vi "Dequeue.vi"(8 "error in (no error)":errorcluster, 11 "Queue In":T1) -> (0 "error out":errorcluster, 1 "Variant":variant, 2 "String":string, 3 "Queue Out":T1)   [LabVIEW 2023, in "Internal Communication.lvlib"]
uses:
  Internal Communication.lvlib
  Controls/Queue.ctl
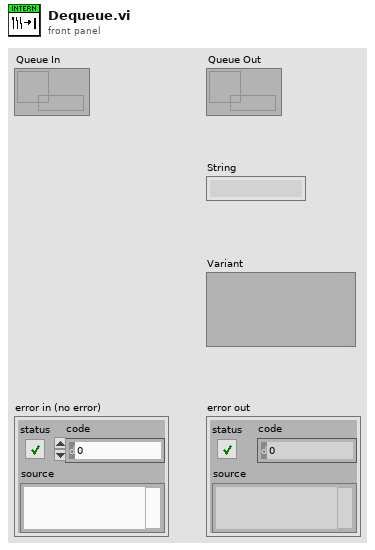
[diagram p1: front panel]
types:
  T1 = typedef "Queue.ctl" = refnum<queue>
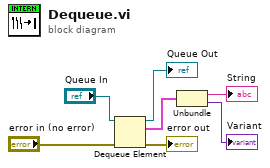
[diagram p0: block diagram]
diagram:
  n1 = Dequeue Element(queue="Queue In", error in (no error)="error in (no error)") -> (queue out=→"Queue Out":T1, element=w4:cluster{string, variant}, error out=→"error out":errorcluster)  [unwired: 1 in, 1 out]
  n2 = Unbundle(w4) -> (→"String":string, →"Variant":variant)
